vi "4-2 matrice 3xM - matrice max - matrice 100x ris2.vi"() -> ()   [LabVIEW 2012]
panel:
  out "B":dbl[](array[numeric]) format="%.2f"
  out "c*(i)":dbl[](array[numeric]) format="%.2f"
  out "A":dbl[](array[numeric]) format="%.2f"
  out "Array":dbl[][](array[numeric]) format="%.2f"
  in  "Numeric":i32=3
  out "a(i)":dbl[](array[numeric]) format="%.2f"
  out "b(i)":dbl[](array[numeric]) format="%.2f"
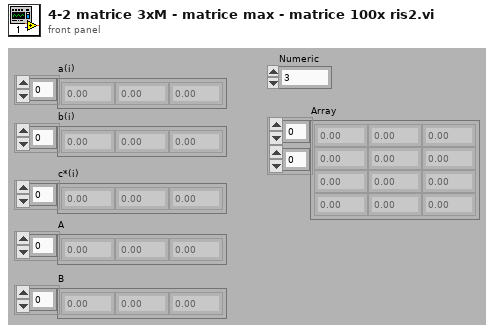
[diagram p1: front panel]
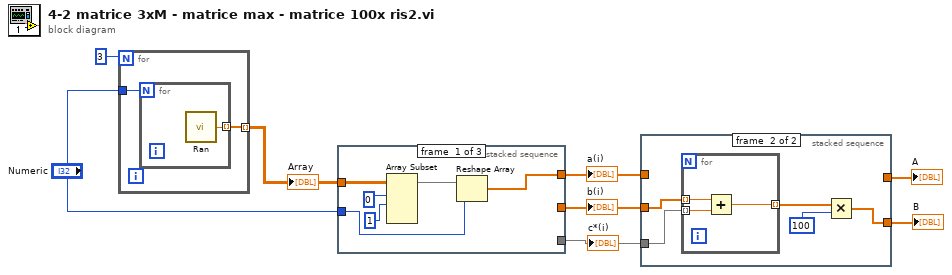
[diagram p0: block diagram]
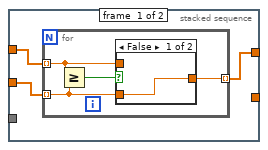
[diagram p2: hidden frame]
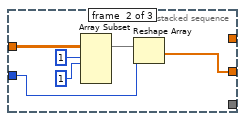
[diagram p4: hidden frame]
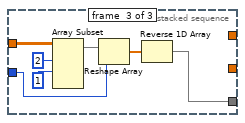
[diagram p5: hidden frame]
diagram:
  n1 = for {
    N: 3 -> [_]
    tunnel: [w10] -> w1 mode=indexing
    tunnel: "Numeric" -> [w9]
    n2 = for {
      N: w9 -> [_]
      tunnel: [w11] -> w10 mode=indexing
      n3 = call "Ran.vi"() -> ("out num"=w11:dbl)  [unwired: 5 in]
    }
  }
  "Array" <- w1
  n4 = stacked-sequence {
    tunnel: w1 -> [w14 w20 w26]
    tunnel: [w13 _ _] -> w7
    tunnel: [_ w19 _] -> w6
    tunnel: [_ _ w25] -> w5
    tunnel: "Numeric" -> [w12 w18 w24]
    frame #0 {
      n5 = Array Subset(array=w14, index (row)=0, length (row)=1) -> (w15:dbl[][])  [unwired: 2 in]
      n6 = Reshape Array(w15, w12) -> (w13:dbl[])
    }
    frame #1 {
      n7 = Array Subset(array=w20, index (row)=1, length (row)=1) -> (w23:dbl[][])  [unwired: 2 in]
      n8 = Reshape Array(w23, w18) -> (w19:dbl[])
    }
    frame #2 {
      n9 = Array Subset(array=w26, index (row)=2, length (row)=1) -> (w29:dbl[][])  [unwired: 2 in]
      n10 = Reshape Array(w29, w24) -> (w30:dbl[])
      n11 = Reverse 1D Array(array=w30) -> (reversed array=w25:dbl[])
    }
  }
  "b(i)" <- w6
  "a(i)" <- w7
  "c*(i)" <- w5
  n12 = stacked-sequence {
    tunnel: w7 -> [w33 _]
    tunnel: w6 -> [w32 w41]
    tunnel: w5 -> [_ w42]
    tunnel: [_ w40] -> w4
    tunnel: [w31 _] -> w3
    frame #0 {
      n13 = for {
        tunnel: w33 -> [w35] mode=indexing
        tunnel: w32 -> [w34] mode=indexing
        tunnel: [w36] -> w31 mode=indexing
        n14 = Greater Or Equal?(x=w35, y=w34) -> (x >= y?=w37:bool)
        n15 = case shown="False" w37 {
          tunnel: [w38 w39] -> w36
          tunnel: w35 -> [_ w39]
          tunnel: w34 -> [w38 _]
          frame False {
          }
          frame True {
          }
        }
      }
    }
    frame #1 {
      n16 = for {
        tunnel: [w47] -> w43 mode=indexing
        tunnel: w42 -> [w46] mode=indexing
        tunnel: w41 -> [w45] mode=indexing
        n17 = Add(x=w45, y=w46) -> (x+y=w47:dbl)
      }
      n18 = Multiply(x=w43, y=100) -> (x*y=w40:dbl[])
    }
  }
  "A" <- w3
  "B" <- w4
